vi "Read Rx Duration.vi"(8 "error in (no error)":errorcluster, 11 "Framework Performance in":refnum<class "Performance.lvclass">) -> (0 "error out":errorcluster, 2 "rx duration":u32 format="%d us", 3 "Framework Performance out":refnum<class "Performance.lvclass">)   [LabVIEW 2017, in "DSF Core.lvlib" / "Performance.lvclass"]
uses:
  Performance.lvclass
  Performance.lvclass/Performance.ctl
  <vilib>/NI/Memory Manager/Classes/Pointer/Pointer.lvclass/Pointer.ctl
  <vilib>/NI/Memory Manager/Classes/Pointer/Get Address.vi
  <vilib>/NI/Memory Manager/Classes/Pointer/Check Null Pointer.vi
  <vilib>/NI/Memory Manager/Classes/Pointer/Check Size (0D).vi
  Timing Status/Timing Status Size.vi
  <vilib>/NI/Memory Manager/Classes/Pointer/Errors.vi
  <vilib>/NI/Memory Manager/Classes/Pointer/Null Pointer.vi
  <vilib>/NI/Memory Manager/Classes/Pointer/Is Null.vi
  <vilib>/NI/Memory Manager/Classes/Pointer/Out of Bounds.vi
  <vilib>/NI/Memory Manager/Classes/Pointer/Get Size.vi
  <vilib>/NI/Memory Manager/Classes/Pointer/Create Error.vi
  <vilib>/NI/Memory Manager/VIs/Source.Write.String.vi
  <vilib>/NI/Memory Manager/Classes/Pointer/Write Pointer Size.vi
  <vilib>/NI/Memory Manager/VIs/Source.Write.Scalar.Base10.vi
  <vilib>/NI/Memory Manager/VIs/Source.Write.Scalar.Base10 (U64).vi
  <vilib>/NI/Memory Manager/VIs/New Error Cluster Constant.vi
  <vilib>/NI/Memory Manager/VIs/New Error Cluster Constant (512B).vi
  <vilib>/NI/Memory Manager/VIs/Error Cluster.Set Status.vi
  <vilib>/NI/Memory Manager/VIs/Error Cluster.Set Code.vi
  <vilib>/NI/Memory Manager/VIs/Error Cluster.Set VI Source.vi
  <vilib>/NI/Memory Manager/Constants/Constants.vi
  <vilib>/NI/Memory Manager/Constants/Library Name.vi
  <vilib>/NI/Memory Manager/Classes/Pointer/Pointer Error Info.vi
  <vilib>/NI/Memory Manager/Constants/Pointer Class Name.vi
  Timing Status/Timing Status.lvclass
  C:/Program Files (x86)/National Instruments/LabVIEW 2017/vi.lib/NI/Memory Manager/Classes/Pointer/Pointer.lvclass
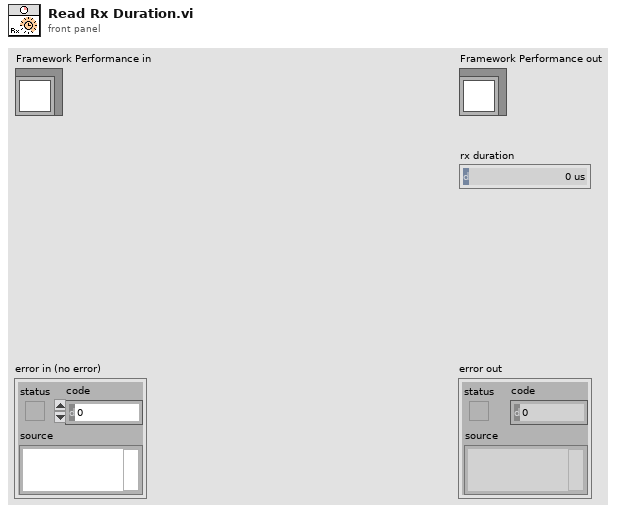
[diagram p1: front panel]
types:
  T1 = typedef "DSF Core.lvlib/Timing Status.lvclass/Timing Status Data.ctl" = cluster{"rx start time":u32, "rx end time":u32, "tx start time":u32, "tx end time":u32, "cycle start time":u32, "cycle end time":u32, "prev start time":u32}
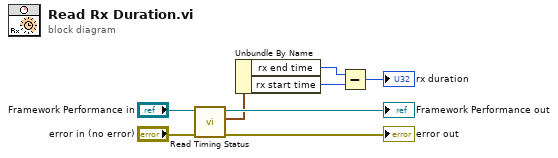
[diagram p0: block diagram]
diagram:
  n1 = call "Read Timing Status.vi"("error in (no error)"="error in (no error)", "Framework Performance in"="Framework Performance in") -> ("error out"=→"error out":errorcluster, "timing status"=w2:T1, "Framework Performance out"=→"Framework Performance out":refnum<class "Performance.lvclass">)  [unwired: 7 in]
  n2 = Unbundle By Name(w2) -> ("rx end time"=w8:u32, "rx start time"=w7:u32)
  n3 = Subtract(x=w8, y=w7) -> (x-y=→"rx duration":u32)
